vi "MsgWriter.vi"() -> ()   [LabVIEW 2020]
panel:
  in  "Test Error code send":errorcluster
  in  "Send Exit Code":bool
  in  "Color":u32(colorbox)
  in  "LineToPrint":string="what hath god wrought"
  in  "Send print line":bool
  out "concatenated string":string
  in  "stop":bool
  out "error out":errorcluster
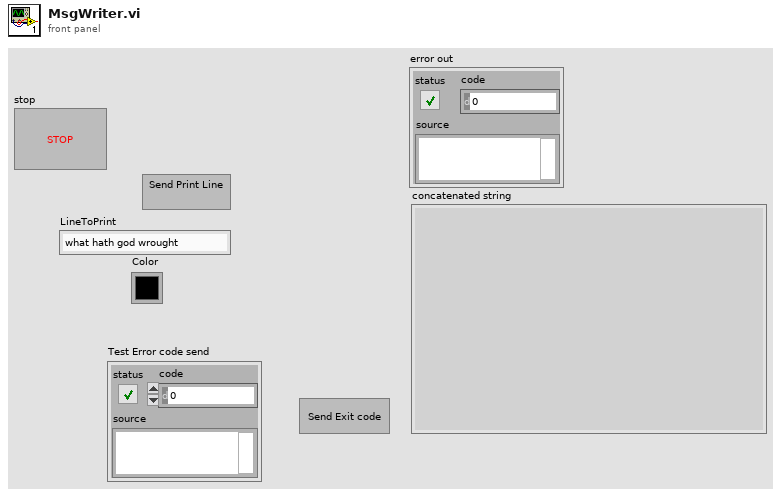
[diagram p1: front panel]
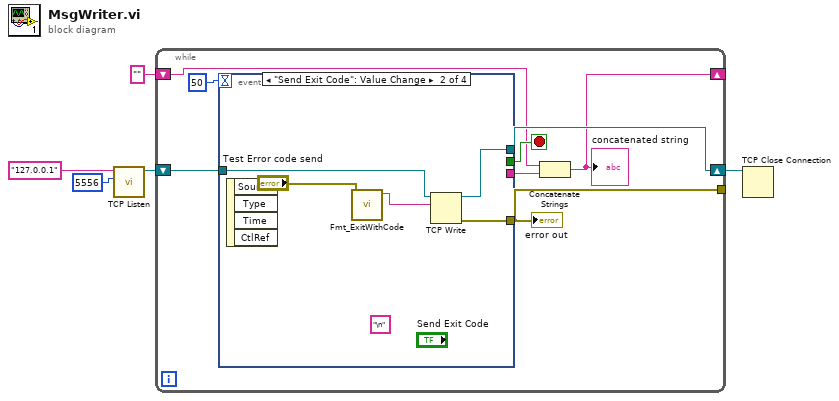
[diagram p0: block diagram]
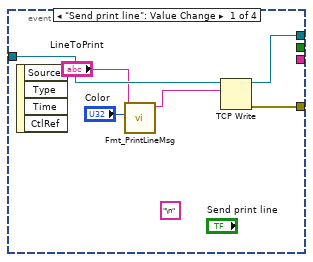
[diagram p2: hidden frame]
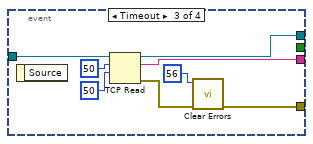
[diagram p3: hidden frame]
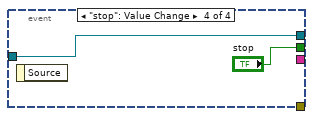
[diagram p4: hidden frame]
diagram:
  n1 = call <vilib>:"TCP Listen.vi"("port"=u16 5556, "service name"="127.0.0.1") -> ("connection ID"=w3:refnum<k5>)  [unwired: 5 in, 4 out]
  n2 = while {
    tunnel: [w12] -> _
    shift-right: [w10] -> w2
    shift-left: w3 -> [w13]
    shift-right: [w8] -> _
    shift-left: "" -> [w7]
    stop <- w11 stop-if-true
    n3 = event shown="[1] \"Send Exit Code\": Value Change" {
      selector: _ -> [_ _ _ _]
      dyn-events: _ -> [_ _ _ _]
      timeout: 50 -> [_ _ _ _]
      tunnel: w13 -> [w19 w22 w32 w33]
      tunnel: [w18 w24 w30 _] -> w12
      tunnel: [_ _ _ "stop"] -> w11
      tunnel: [w17 w23 w27 w33] -> w10
      tunnel: [_ _ w26 _] -> w9
      event "Send print line": Value Change {
        (unwired) "\n" ("string")
        n4 = event-data() -> ()  [unwired: 1 in, 4 out]
        n5 = call "Fmt_PrintLineMsg.vi"("Color"="Color", "LineToPrint"="LineToPrint") -> ("<JSON>"=w14:string)  [unwired: 9 in]
        n6 = TCP Write(connection ID=w19, data in=w14) -> (connection ID out=w17:refnum<k5>, error out=w18:errorcluster)  [unwired: 2 in, 1 out]
      }
      event "Send Exit Code": Value Change {
        (unwired) "\n" ("string")
        n7 = event-data() -> ()  [unwired: 1 in, 4 out]
        n8 = call "Fmt_ExitWithCode.vi"("error in (no error)"="Test Error code send") -> ("<JSON>"=w21:string)  [unwired: 10 in]
        n9 = TCP Write(connection ID=w22, data in=w21) -> (connection ID out=w23:refnum<k5>, error out=w24:errorcluster)  [unwired: 2 in, 1 out]
      }
      event Timeout {
        n10 = event-data() -> ()  [unwired: 1 in, 1 out]
        n11 = TCP Read(connection ID=w32, bytes to read=50, 9:50 ("timeout ms (25000)")) -> (connection ID out=w27:refnum<k5>, data out=w26:string, error out=w28:errorcluster)  [unwired: 2 in]
        n12 = call <vilib>:"Clear Errors.vi"("error in (no error)"=w28, "specific error code to clear (0: all)"=56) -> ("error out"=w30:errorcluster)  [unwired: 4 in, 1 out]
      }
      event "stop": Value Change {
        n13 = event-data() -> ()  [unwired: 1 in, 1 out]
      }
    }
    "error out" <- w12
    n14 = Concatenate Strings(w7, w9) -> (w8:string)
    "concatenated string" <- w8
  }
  n15 = TCP Close Connection(connection ID=w2) -> ()  [unwired: 2 in, 2 out]
